vi "Global Position to Pixel.vi"(7 "picture info":T1={"picture size"={"Width"=500, "Height"=500}, "pixels per unit"=10.0}, 10 "global y":dbl, 11 "global x":dbl) -> (2 "pixel y":i16, 3 "pixel x":i16)   [LabVIEW 2017, in "NI_Robotics_Steering Picture.lvlib"]
uses:
  <vilib>/robotics/Utilities/Visualization/Steering Visualization/Steering Picture/NI_Robotics_Steering Picture.lvlib
  <vilib>/robotics/Utilities/Visualization/Steering Visualization/Steering Picture/Picture Info.ctl
  <vilib>/Utility/miscctls.llb/LVBoundsTypeDef.ctl
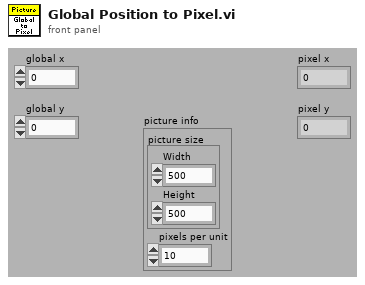
[diagram p1: front panel]
types:
  T1 = typedef "NI_Robotics_Steering Picture.lvlib/Picture Info.ctl" = cluster{"picture size":T2, "pixels per unit":dbl}
  T2 = typedef "LVBoundsTypeDef.ctl" = cluster{"Width":u32, "Height":u32}
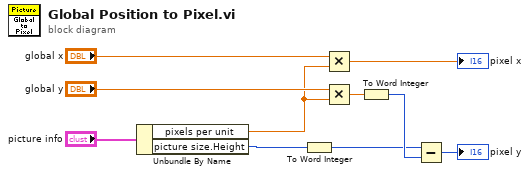
[diagram p0: block diagram]
diagram:
  n1 = Unbundle By Name("picture info") -> ("pixels per unit"=w3:dbl, "picture size.Height"=w2:u32)
  n2 = To Word Integer(number=w2) -> (16bit integer=w1:i16)
  n3 = Multiply(x="global x", y=w3) -> (x*y=→"pixel x":dbl)
  n4 = Multiply(x="global y", y=w3) -> (x*y=w7:dbl)
  n5 = To Word Integer(number=w7) -> (16bit integer=w5:i16)
  n6 = Subtract(x=w1, y=w5) -> (x-y=→"pixel y":i16)
